vi "Ramsete_Execute_ENG.vi"(4 "Enabled":bool=TRUE, 6 "Reset":bool, 7 "RAMSETE_EXE_TUNING":T4={"B"=2.0, "Zeta"=0.7, "X Tolerance M"=2.0, "Y Tolerance M"=0.7, "Heading Tolerance RAD"=0.7, "Track Width M"=2.0, "Max Speed M/S"=2.0} {"Max Speed M/S" format="%13.4f"; "Track Width M" format="%13.4f"; "Heading Tolerance RAD" format="%13.4f"; "Y Tolerance M" format="%13.4f"; "X Tolerance M" format="%13.4f"; "Zeta" format="%13.4f"; "B" format="%13.4f"}, 8 "Gyro-Deg\n(Inc counterclockwise)":dbl, 9 "RightDist-Ft":dbl, 10 "LeftDist-Ft":dbl, 11 "TRAJ_STATE  SI":T6 {"POSE"."ROTATION"."SIN" format="%13.4f"; "POSE"."ROTATION"."COS" format="%13.4f"; "POSE"."ROTATION"."VALUE" format="%13.4f"; "POSE"."TRANSLATION"."Y" format="%14.3f"; "POSE"."TRANSLATION"."X" format="%14.3f"}) -> (0 "CurrentRelativePose ENG":T1 {"ROTATION"."SIN" format="%13.4f"; "ROTATION"."COS" format="%13.4f"; "ROTATION"."VALUE" format="%13.4f"; "TRANSLATION"."Y" format="%14.3f"; "TRANSLATION"."X" format="%14.3f"}, 1 "AtReference":bool, 2 "Right Speed Dmd Ft/S":dbl, 3 "Left Speed Dmd Ft/S":dbl, 5 "outRAMSETE":T5={"B"=2.0, "Zeta"=0.7, "poseTolerance"={"TRANSLATION"={"X"=0.0, "Y"=0.0}, "ROTATION"={"VALUE"=0.0, "COS"=1.0, "SIN"=0.0}}, "poseError"={"TRANSLATION"={"X"=0.0, "Y"=0.0}, "ROTATION"={"VALUE"=0.0, "COS"=1.0, "SIN"=0.0}}, "Enabled"=TRUE} {"poseError"."ROTATION"."SIN" format="%13.4f"; "poseError"."ROTATION"."COS" format="%13.4f"; "poseError"."ROTATION"."VALUE" format="%13.4f"; "poseError"."TRANSLATION"."Y" format="%14.3f"; "poseError"."TRANSLATION"."X" format="%14.3f"; "poseTolerance"."ROTATION"."SIN" format="%13.4f"; "poseTolerance"."ROTATION"."COS" format="%13.4f"; "poseTolerance"."ROTATION"."VALUE" format="%13.4f"; "poseTolerance"."TRANSLATION"."Y" format="%14.3f"; "poseTolerance"."TRANSLATION"."X" format="%14.3f"; "Zeta" format="%12.3f"; "B" format="%12.3f"})   [LabVIEW 2019, in "Trajectory_Library.lvlib"]
doc: "Convienience function to create and calculate the ramsete control, returning normalized desired left and right speed setpoints \n\nThis is designed for ENG units -- Feet, degrees.\n\n\nParameters: \n - Ramsete EXE Tuning -- Packed data cluster containing the ramsete tuning parameters and Differntial Drive kinematics information.\n - TrajState - Desired trajectory state\n - Left Dist -- The left distance read from encoders (Feet). The encoders do NOT have to be reset at the beginning of trajectory execution.\n - Right Dist -- The right distance read from encoders (Feet). The encoders do NOT have to be reset at the beginning of trajectory execution.\n - Gyro - The current reading of a gyro whose value increases counter clockwise. (You may need to negate your gyro reading.) (Degrees)\n - Reset -- Resets the current robot pose and the beginning left and right distances and the gyro reading\n - Enabled -- When enabled uses the ramsete closed loop control to drive the left and right speed demand outputs. When disabled the trajectory data is directly converted to left and right speed demands.\n\n\nReturns:\n - Left Speed Dmd -- Left Speed demand (Feet/Second)\n - Right Speed Dmd -- Right Speed demand (Feet/Second)\n - Out Ramsete -- Updated Ramsete data structure\n - Current Relative Pose -- Current robot relative pose. This pose is reset to zero when the RESET input is set to TRUE. \n - At Reference -- Set to TRUE when the current robot pose is withing the specified tolerance of the desired POSE from the trajectory state input."
uses:
  Trajectory_Library.lvlib
  TypeDef/TRAJ_STATE.ctl
  TypeDef/POSE2D.ctl
  TypeDef/TRANSLATION2D.ctl
  TypeDef/ROTATION2D.ctl
  TypeDef/RAMSETE.ctl
  TypeDef/RAMSETE_EXE_TUNING.ctl
  Ramsete_New_B_Z.vi
  Ramsete_SetTolerance.vi
  Pose2d_New.vi
  Conv_AngleRadians_Heading.vi
  Ramsete_SetEnabled.vi
  Conv_Radians_Deg.vi
  Rotation2d_CreateAngle.vi
  Translation2d_Create.vi
  Ramsete_Diff_DO_SI.vi
  DiffWheel_Normalize.vi
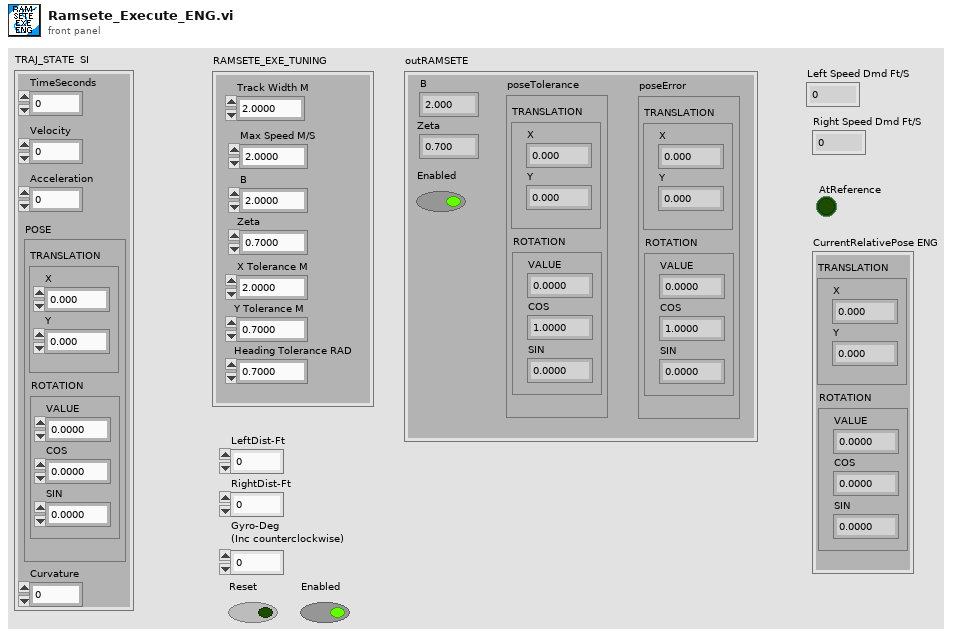
[diagram p1: front panel]
types:
  T1 = typedef "Trajectory_Library.lvlib/POSE2D.ctl" = cluster{"TRANSLATION":T2, "ROTATION":T3}
  T2 = typedef "Trajectory_Library.lvlib/TRANSLATION2D.ctl" = cluster{"X":dbl, "Y":dbl}
  T3 = typedef "Trajectory_Library.lvlib/ROTATION2D.ctl" = cluster{"VALUE":dbl, "COS":dbl, "SIN":dbl}
  T4 = typedef "Trajectory_Library.lvlib/RAMSETE_EXE_TUNING.ctl" = cluster{"B":dbl, "Zeta":dbl, "X Tolerance M":dbl, "Y Tolerance M":dbl, "Heading Tolerance RAD":dbl, "Track Width M":dbl, "Max Speed M/S":dbl}
  T5 = typedef "Trajectory_Library.lvlib/RAMSETE.ctl" = cluster{"B":dbl, "Zeta":dbl, "poseTolerance":T1, "poseError":T1, "Enabled":bool}
  T6 = typedef "Trajectory_Library.lvlib/TRAJ_STATE.ctl" = cluster{"TimeSeconds":dbl, "Velocity":dbl, "Acceleration":dbl, "POSE":T1, "Curvature":dbl}
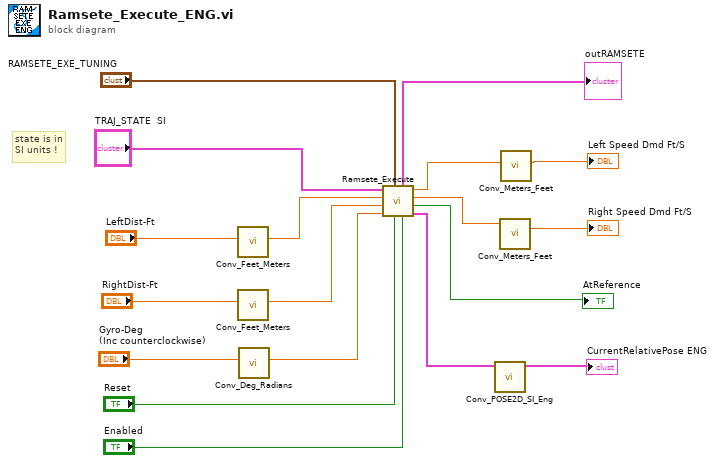
[diagram p0: block diagram]
diagram:
  # "state is in\nSI units !"
  n1 = call "Conv_Feet_Meters.vi"("Feet"="LeftDist-Ft") -> ("Meters"=w13:dbl)  [unwired: 10 in]
  n2 = call "Conv_Feet_Meters.vi"("Feet"="RightDist-Ft") -> ("Meters"=w12:dbl)  [unwired: 10 in]
  n3 = call "Conv_Deg_Radians.vi"("Degress"="Gyro-Deg\n(Inc counterclockwise)") -> ("Radians"=w11:dbl)  [unwired: 10 in]
  n4 = call "Ramsete_Execute.vi"("Enabled"="Enabled", "Reset"="Reset", "RAMSETE_EXE_TUNING"="RAMSETE_EXE_TUNING", "Gyro-Radians\n(Inc counterclockwise)"=w11, "RightDist-Meters"=w12, "LeftDist-Meters"=w13, "TRAJ_STATE"="TRAJ_STATE  SI") -> ("CurrentRelativePose"=w6:T1, "AtReference"=→"AtReference":bool, "Right Speed Dmd M/S"=w5:dbl, "Left Speed Dmd M/S"=w8:dbl, "outRAMSETE"=→"outRAMSETE":T5)
  n5 = call "Conv_POSE2D_SI_Eng.vi"("Err Pose in SI"=w6) -> ("Err Pose out ENG"=→"CurrentRelativePose ENG":T1)  [unwired: 10 in]
  n6 = call "Conv_Meters_Feet.vi"("Meters"=w5) -> ("Feet"=→"Right Speed Dmd Ft/S":dbl)  [unwired: 10 in]
  n7 = call "Conv_Meters_Feet.vi"("Meters"=w8) -> ("Feet"=→"Left Speed Dmd Ft/S":dbl)  [unwired: 10 in]
